vi "session_methods.vi"() -> ()   [LabVIEW 2017]
doc: "Illustrates how to configure preferred methods and return the negotiated methods."
uses:
  libssh2/libssh2_method_type.ctl
  libssh2/libssh2_flag.ctl
  libssh2/libssh2_session_handshake_tcp.vi
  libssh2/libssh2_init_default.vi
  libssh2/libssh2_session_init_ex.vi
  <vilib>/Utility/tcp.llb/TCP Get Raw Net Object.vi
  libssh2/libssh2_session_handshake_socket.vi
  libssh2/libssh2.lvlib
panel:
  out "supported algorithms":cluster{"method_type":T1, "algs":string[]}[](array[cluster])
  in  "method preferences":cluster{"method_type":T1, "prefs":string}[](array[cluster])=[{"method_type"=enum."LIBSSH2_METHOD_KEX", "prefs"="curve25519-sha256"}]
  out "negotiated methods":cluster{"method_type":T1, "methods":string}[](array[cluster])
  in  "method_type (hidden)":T1
  out "error out":errorcluster
  in  "hostname":string="localhost"
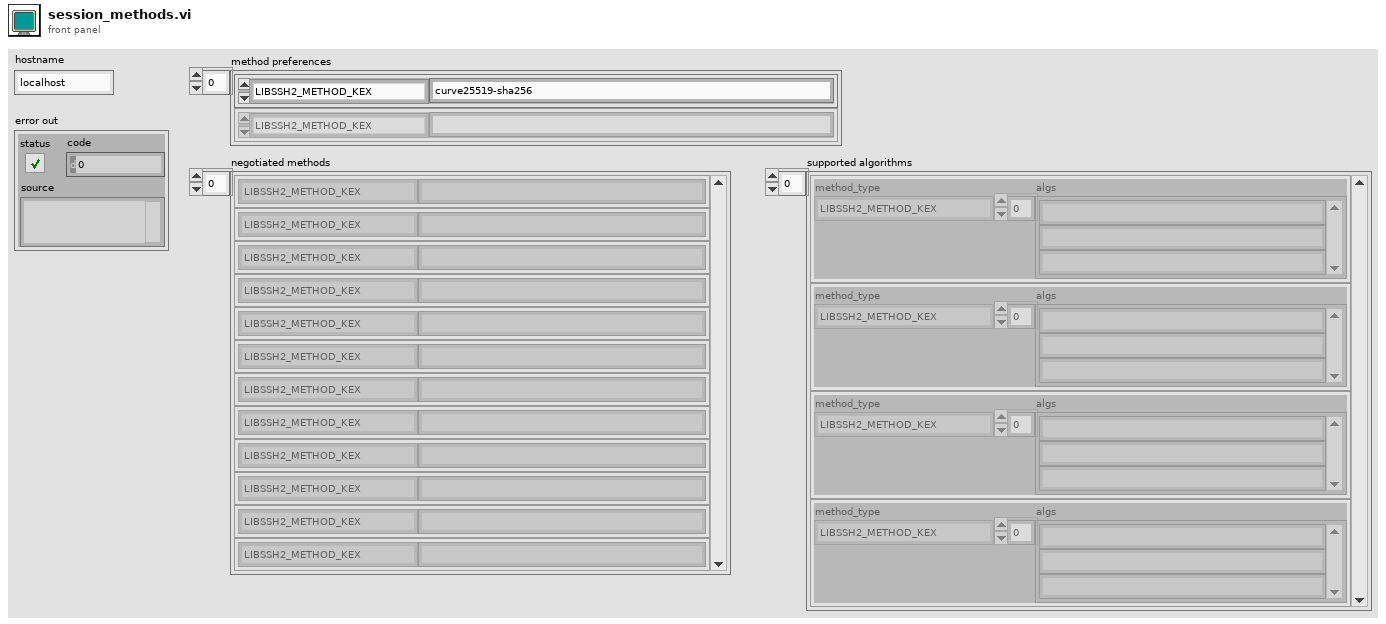
[diagram p1: front panel]
types:
  T1 = typedef "libssh2.lvlib/libssh2_method_type.ctl" = enum16{"LIBSSH2_METHOD_KEX", "LIBSSH2_METHOD_HOSTKEY", "LIBSSH2_METHOD_CRYPT_CS", "LIBSSH2_METHOD_CRYPT_SC", "LIBSSH2_METHOD_MAC_CS", "LIBSSH2_METHOD_MAC_SC", "LIBSSH2_METHOD_COMP_CS", "LIBSSH2_METHOD_COMP_SC", "LIBSSH2_METHOD_LANG_CS", "LIBSSH2_METHOD_LANG_SC", "LIBSSH2_METHOD_SIGN_ALGO"}
  T2 = typedef "libssh2.lvlib/libssh2_flag.ctl" = enum16{"SIGPIPE", "COMPRESS", "QUOTE_PATHS"}
  T3 = typedef "libssh2.lvlib/Session Refnum.ctl" = refnum<k1>
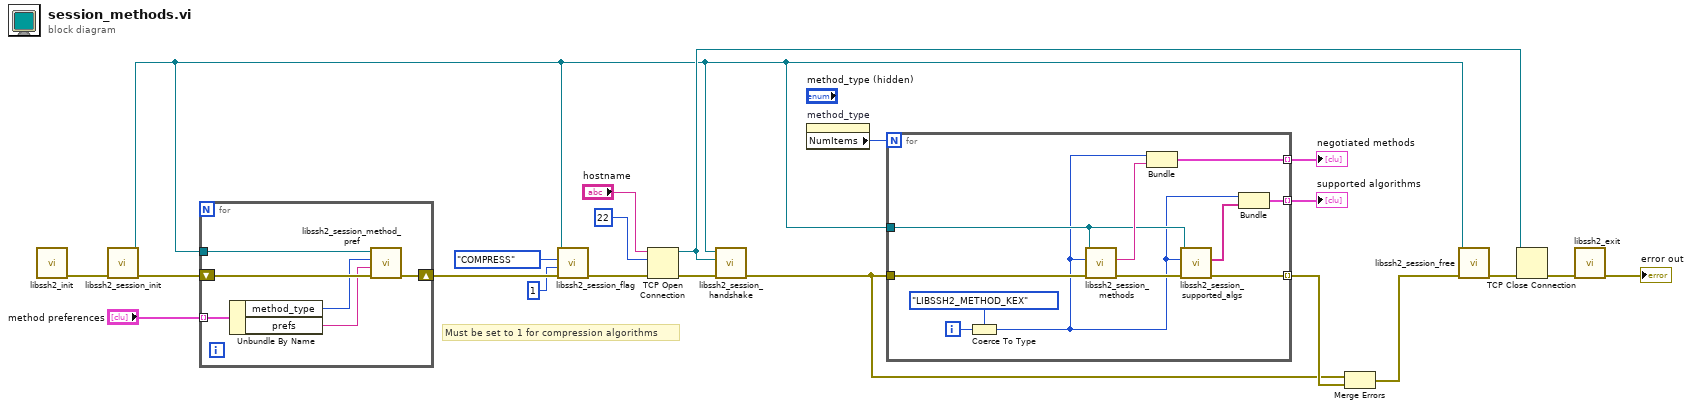
[diagram p0: block diagram]
diagram:
  # "Must be set to 1 for compression algorithms"
  n1 = call-poly "libssh2_init.vi"() -> ("error out"=w21:errorcluster)  [unwired: 11 in]
  n2 = call "libssh2_session_init.vi"("error in (no error)"=w21) -> ("error out"=w14:errorcluster, "session"=w5:T3)  [unwired: 9 in]
  n3 = for {
    tunnel: w5 -> [w25]
    shift-right: [w26] -> w10
    shift-left: w14 -> [w27]
    tunnel: "method preferences" -> [w24] mode=indexing
    n4 = Unbundle By Name(w24) -> ("method_type"=w23:T1, "prefs"=w22:string)
    n5 = call "libssh2_session_method_pref.vi"("error in (no error)"=w27, "prefs"=w22, "method_type"=w23, "session"=w25) -> ("error out"=w26:errorcluster)  [unwired: 7 in]
  }
  n6 = call "libssh2_session_flag.vi"("error in (no error)"=w10, "value (0 = disabled)"=1, "flag"=libssh2_flag."COMPRESS", "session"=w5) -> ("error out"=w6:errorcluster)  [unwired: 7 in]
  n7 = TCP Open Connection(address="hostname", remote port or service name=u16 22, error in (no error)=w6) -> (connection ID=w15:refnum<k5>, error out=w16:errorcluster)  [unwired: 2 in]
  n8 = call-poly "libssh2_session_handshake.vi"("error in (no error)"=w16, "tcp connection"=w15, "session"=w5) -> ("error out"=w7:errorcluster)  [unwired: 8 in]
  n9 = property on="method_type" class="Enum (strict)"() -> ("NumItems"=w2:u32)  [unwired: 2 in, 2 out]
  n10 = for {
    N: w2 -> [_]
    tunnel: w5 -> [w31]
    tunnel: [w33] -> w12 mode=indexing
    tunnel: w7 -> [w38]
    tunnel: [w32] -> w11 mode=indexing
    tunnel: [w28] -> w1 mode=indexing
    i -> [w36]
    n11 = Coerce To Type(0:w36, 1:libssh2_method_type."LIBSSH2_METHOD_KEX" ("method_type")) -> (2:w30:T1)
    n12 = call "libssh2_session_methods.vi"("error in (no error)"=w38, "method_type"=w30, "session"=w31) -> ("error out"=w37:errorcluster, "methods"=w34:string)  [unwired: 7 in]
    n13 = Bundle("method_type"=w30, "methods"=w34) -> (w33:cluster{"method_type":T1, "methods":string})  [unwired: 1 in]
    n14 = call "libssh2_session_supported_algs.vi"("error in (no error)"=w37, "method_type"=w30, "session"=w31) -> ("error out"=w32:errorcluster, "algs"=w29:string[])  [unwired: 7 in]
    n15 = Bundle("method_type"=w30, "algs"=w29) -> (w28:cluster{"method_type":T1, "algs":string[]})  [unwired: 1 in]
  }
  "negotiated methods" <- w12
  "supported algorithms" <- w1
  n16 = Merge Errors(w7, w11) -> (w8:errorcluster)
  n17 = call "libssh2_session_free.vi"("error in (no error)"=w8, "session"=w5) -> ("error out"=w20:errorcluster)  [unwired: 9 in]
  n18 = TCP Close Connection(connection ID=w15, error in (no error)=w20) -> (error out=w17:errorcluster)  [unwired: 1 in, 1 out]
  n19 = call "libssh2_exit.vi"("error in (no error)"=w17) -> ("error out"=→"error out":errorcluster)  [unwired: 10 in]
